vi "GetTACWindow.vi"(0 "Enum":enum16{"ini", "get", "quick"}(ring), 4 "auto":bool) -> (1 "TAC.Window (diff)":u16, 2 "Waveform Graph 2":refnum<vi>, 3 "Decays":u32[][](graph), 5 "TAC.Window (min)":u16, 6 "allchan?":bool, 7 "Cursor.Cursor Position:Cursor X":u16, 8 "Cursor.Cursor Position:Cursor X 2":u16, 9 "x-values":dbl[](array[numeric]) format="%.2f", 10 "ready?":bool)   [LabVIEW 2009]
uses:
  IMAGE Cluster 2.ctl
panel:
  out "rebinning":dbl
  out "TAC Range (ns)":sgl
  in  "ADC-Resolution":u16(ring) items=["8bit", "12bit", "4bit", "15bit"]
  in  "Ring":u8(ring)=1 items=["linear y-axis", "log y-axis"]
  out "Boolean 2":bool
  in  "TAC-Cube (for Spotfinder)":T1(ring)=enum."no Spotfinding"
  in  "OK Button":bool
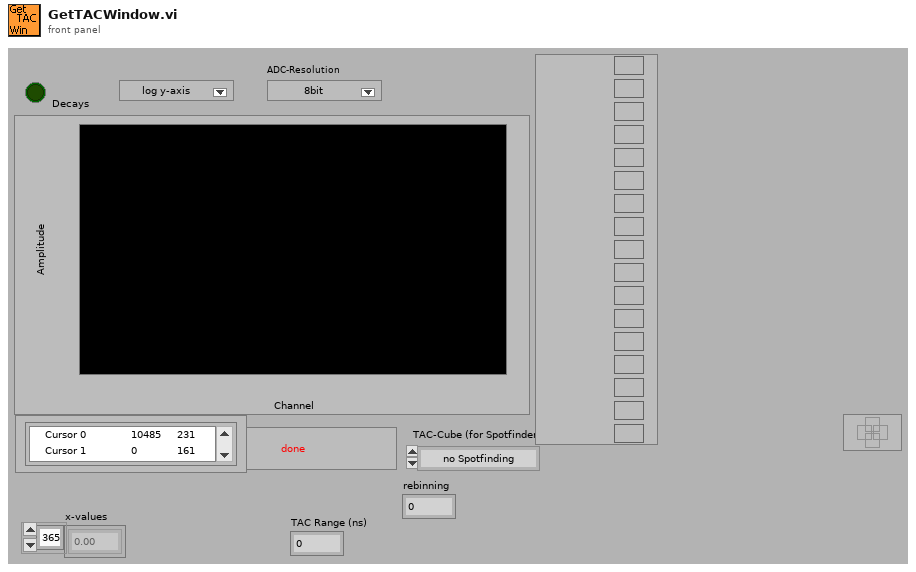
[diagram p1: front panel]
types:
  T1 = enum16{"1", "2", "3", "4", "5", "6", "7", "Sum", "no Spotfinding", "Separation"}
  T2 = typedef "IMAGE Cluster 2.ctl" = cluster{"decay":u16[][][][][], "sum of photons":u32[][][][]}
  T3 = typedef "FIFOSettings_BH.ctt" = cluster{"Measurement":cluster{"Binning (ms)":sgl, "External Trigger Condition":u16, "Stop Condition:":u16, "Stop Count":dbl, "Buffer Size (Photons)":u16, "No of Channels":u16, "Ext Latch Delay":i16}, "ADC":cluster{"Module":u16, "ADC Resolution":i32, "Dither Range":i16, "Count Increment":i16, "Macro Time Clock":i16}, "SYNC":cluster{"SYNC ZC Level (mV)":sgl, "SYNC Freq Divider":i16, "SYNC Holdoff (ns)":sgl, "SYNC Threshold (mV)":sgl}, "TAC":cluster{"TAC Range (ns)":sgl, "TAC Gain":i16, "TAC Offset (%)":sgl, "TAC Limit Low (%)":sgl, "TAC Limit High (%)":sgl}, "CFD":cluster{"CFD Limit Low (mV)":sgl, "CFD Limit High (mV)":sgl, "CFD ZC Level (mV)":sgl, "CFD Holdoff (ns)":sgl}}
  T4 = typedef "Settings.ctl" = cluster{"threshold":cluster{"max":u32, "min":u32}, "RGB or false color":bool, "16bit":bool, "log/lin axis":u16, "spotsize button":bool, "Pixelsize":u16, "autoscale x":bool, "autoscale y":bool, "correlation":bool, "ADC-Resolution":i32, "F2-lifetime":cluster{"display tau":bool, "display F2":bool, "Palette Number lifetime":enum32{"Gray", "Binary", "Gradient", "Rainbow", "Temperature"}, "Palette Number F2":enum32{"Gray", "Binary", "Gradient", "Rainbow", "Temperature"}, "max tau-Value":dbl, "min tau-Value":dbl, "max F2-Value":dbl, "min F2-Value":dbl}, "TAC-Window 1":u16, "TAC-Window 2":u16, "false color palette":cluster{"1":u32, "2":u32, "3":u32, "4":u32, "5":u32, "6":u32, "7":u32, "8":u32, "8 2":u32, "8 3":u32, "8 4":u32, "8 5":u32}, "rebinning":dbl}
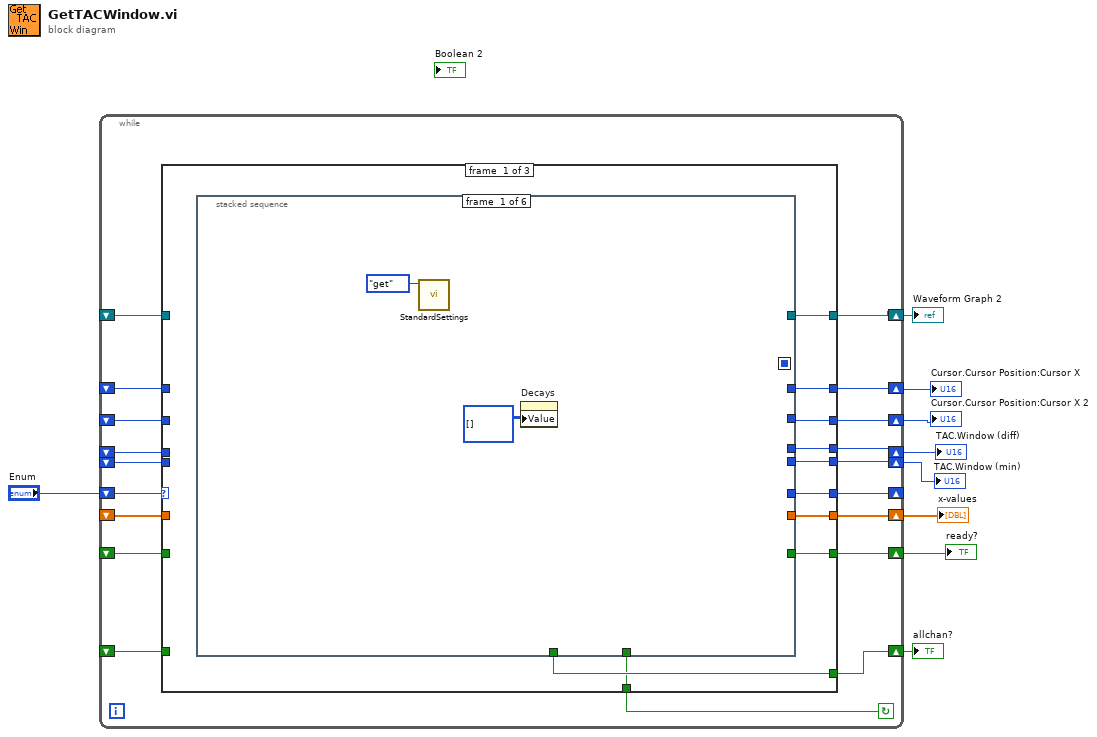
[diagram p0: block diagram]
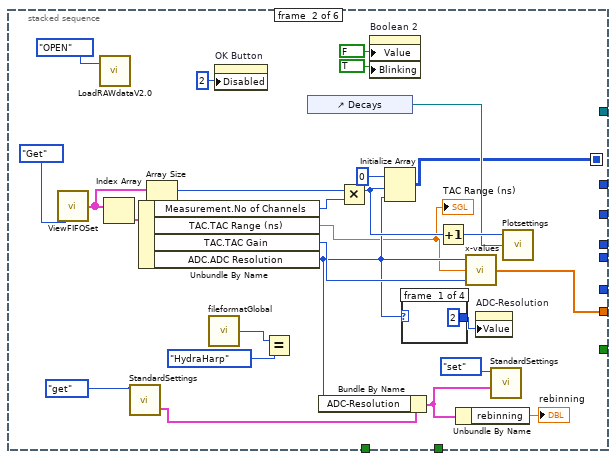
[diagram p2: hidden frame]
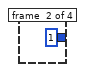
[diagram p3: hidden frame]
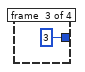
[diagram p4: hidden frame]
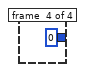
[diagram p5: hidden frame]
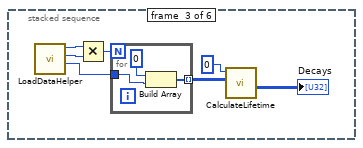
[diagram p6: hidden frame]
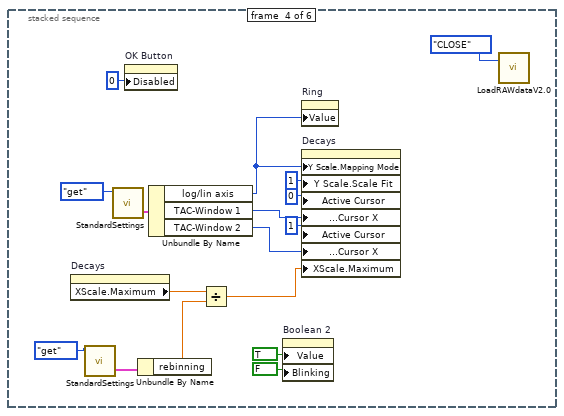
[diagram p7: hidden frame]
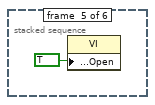
[diagram p8: hidden frame]
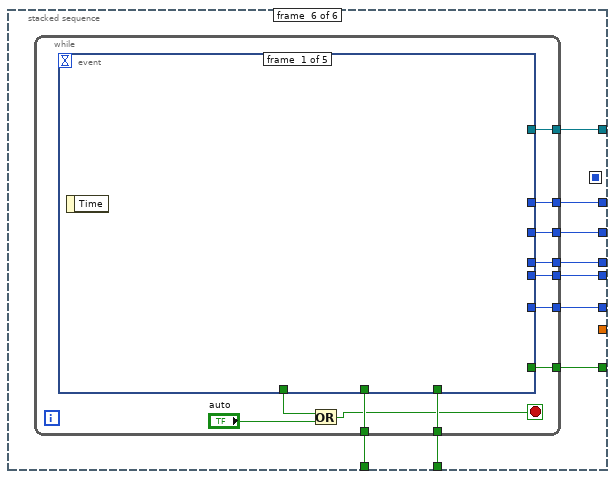
[diagram p9: hidden frame]
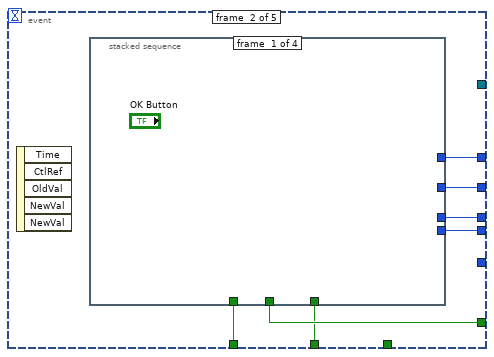
[diagram p10: hidden frame]
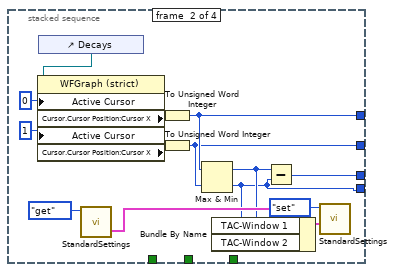
[diagram p11: hidden frame]
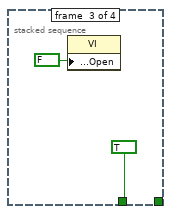
[diagram p12: hidden frame]
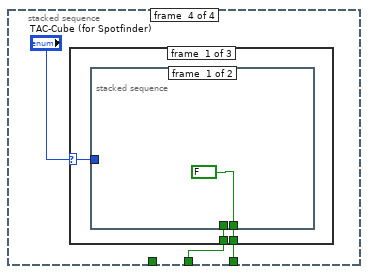
[diagram p13: hidden frame]
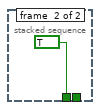
[diagram p14: hidden frame]
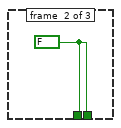
[diagram p15: hidden frame]
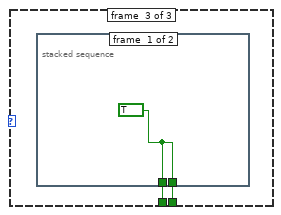
[diagram p16: hidden frame]
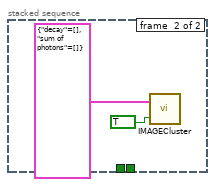
[diagram p17: hidden frame]
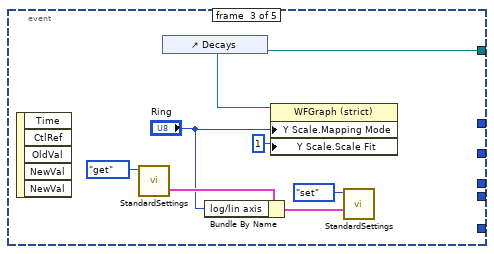
[diagram p18: hidden frame]
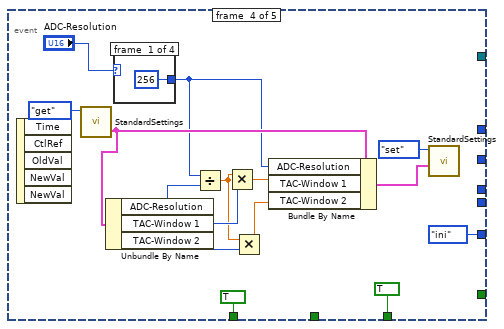
[diagram p19: hidden frame]
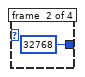
[diagram p20: hidden frame]
diagram:
  n1 = while {
    shift-right: [w28] -> w8
    shift-left: _ -> [w26]
    shift-right: [w27] -> w9
    shift-left: _ -> [w25]
    shift-right: [w24] -> w7
    shift-left: _ -> [w23]
    shift-right: [w21] -> w5
    shift-left: _ -> [w19]
    shift-right: [w22] -> w6
    shift-left: _ -> [w20]
    shift-right: [w13] -> w4
    shift-left: _ -> [w18]
    shift-right: [w17] -> w3
    shift-left: _ -> [w16]
    shift-right: [w15] -> w2
    shift-left: _ -> [w14]
    shift-right: [w10] -> _
    shift-left: "Enum" -> [w11]
    stop <- w12 continue-if-true
    n2 = case shown="\"ini\", Default" w11 {
      tunnel: [w38 w191 w205] -> w28
      tunnel: [w37 w190 w204] -> w27
      tunnel: w26 -> [_ w191 _]
      tunnel: w25 -> [_ w190 _]
      tunnel: [w36 w189 w193] -> w24
      tunnel: w23 -> [_ w189 _]
      tunnel: [w35 w188 w210] -> w22
      tunnel: [w34 w187 w211] -> w21
      tunnel: w20 -> [_ w188 w210]
      tunnel: w19 -> [_ w187 w211]
      tunnel: [w33 w186 w212] -> w13
      tunnel: w18 -> [_ w186 w212]
      tunnel: [w32 w185 w209] -> w17
      tunnel: w16 -> [_ w185 w209]
      tunnel: [w31 w184 w208] -> w15
      tunnel: w14 -> [_ w184 w208]
      tunnel: [w30 _ _] -> w12
      tunnel: [w29 _ _] -> w10
      frame #0 {
        n3 = stacked-sequence {
          seq-local: [_ w42 _ _ _ _] -> [_ _ _ _ _ _]
          tunnel: [_ _ _ _ _ w107] -> w38
          tunnel: [_ _ _ _ _ w106] -> w37
          tunnel: [_ w47 _ _ _ _] -> w36
          tunnel: [_ _ _ _ _ w105] -> w35
          tunnel: [_ _ _ _ _ w104] -> w34
          tunnel: [_ _ _ _ _ w103] -> w33
          tunnel: [_ _ _ _ _ w102] -> w32
          tunnel: [_ _ _ _ _ w101] -> w31
          tunnel: [_ _ _ _ _ w100] -> w30
          tunnel: [_ _ _ _ _ w99] -> w29
          frame #0 {
            n4 = call "StandardSettings.vi"("Enum"=enum16{"Load", "get", "Save", "set"}."get") -> ()  [unwired: 4 in, 1 out]
            n5 = property on="Decays" class="WFGraph (strict)"("Value"=u32[][] [] ("Waveform Graph")) -> ()  [unwired: 2 in, 2 out]
          }
          frame #1 {
            n6 = call "ViewFIFOSet.vi"("Enum"=enum16{"Display", "change", "Get", "Set"}."Get") -> ("FIFO Settings (Array)"=w54:T3[])  [unwired: 1 in]
            n7 = call "LoadRAWdataV2.0.vi"("action"=enum16{"OPEN", "READ", "CLOSE"}."OPEN" ("Enum")) -> ()  [unwired: 1 in, 2 out]
            n8 = Index Array(array=w54) -> (element=w55:T3)  [unwired: 1 in]
            n9 = call "StandardSettings.vi"("Enum"=enum16{"Load", "get", "Save", "set"}."get") -> ("StandardSettings"=w46:T4)  [unwired: 4 in]
            n10 = Unbundle By Name(w55) -> ("Measurement.No of Channels"=w53:u16, "TAC.TAC Range (ns)"=w41:sgl, "TAC.TAC Gain"=w61:i16, "ADC.ADC Resolution"=w50:i32)
            "TAC Range (ns)" <- w41
            n11 = Array Size(array=w54) -> (size(s)=w52:i32)
            n12 = call "fileformatGlobal.vi"() -> ("fileformat out"=w49:enum16{"Herty", "Ken", "SPC130", "HydraHarp"})  [unwired: 2 in]
            n13 = property on="OK Button" class="Boolean"("Disabled"=u8 2) -> ()  [unwired: 2 in, 2 out]
            n14 = Equal?(x=w49, y=enum16{"Herty", "Ken", "SPC130", "HydraHarp"}."HydraHarp") -> ()  [unwired: 1 out]
            n15 = control-ref of="Decays"() -> (w56:refnum<vi>)
            n16 = Bundle By Name(cluster=w46, "ADC-Resolution"=w50) -> (w44:T4)
            n17 = Multiply(x=w52, y=w53) -> (x*y=w51:i32)
            n18 = property on="Boolean 2" class="Boolean (strict)"("Value"=FALSE ("Boolean 2"), "Blinking"=TRUE) -> ()  [unwired: 2 in, 2 out]
            n19 = Initialize Array(u32 0 ("element"), w51, w50) -> (w42:u32[][])
            n20 = case shown="32768" w50 {
              tunnel: [u16 2 u16 1 u16 3 u16 0] -> w43
              frame #0 {
              }
              frame #1 {
              }
              frame #2 {
              }
              frame #3 {
              }
            }
            n21 = Increment(x=w51) -> (x+1=w58:i32)
            n22 = Unbundle By Name(w44) -> ("rebinning"=→"rebinning":dbl)
            n23 = call "x-values.vi"("TAC Gain"=w61, "TAC Rang [ns]"=w41, "No. Microchannel"=w50) -> ("Array"=w47:dbl[])
            n24 = property on="ADC-Resolution" class="Ring (strict)"("Value"=w43) -> ()  [unwired: 2 in, 2 out]
            n25 = call "StandardSettings.vi"("StandardSettings"=w44, "Enum"=enum16{"Load", "get", "Save", "set"}."set") -> ()  [unwired: 3 in, 1 out]
            n26 = call "Plotsettings.vi"("Decays 2"=w56, "No of Channels"=w58) -> ()  [unwired: 4 in]
          }
          frame #2 {
            n27 = call "LoadDataHelper.vi"() -> ("pixel per line"=w73:u32, "planes"=w74:u32, "lines"=w75:u32)  [unwired: 7 in, 2 out]
            n28 = Multiply(x=w75, y=w74) -> (x*y=w76:u32)
            n29 = for {
              N: w76 -> [_]
              tunnel: w73 -> [w79]
              tunnel: [w78] -> w72 mode=indexing
              n30 = Build Array(0 ("starting y-point"), w79) -> (w78:u32[])
            }
            n31 = call "CalculateLifetime.vi"("Pos Array"=w72, "starting y-point"=0) -> ("Decay"=→"Decays":u32[][])  [unwired: 5 in]
          }
          frame #3 {
            n32 = property on="Decays" class="WFGraph (strict)"() -> ("XScale.Maximum"=w85:dbl)  [unwired: 2 in, 2 out]
            n33 = call "StandardSettings.vi"("Enum"=enum16{"Load", "get", "Save", "set"}."get") -> ("StandardSettings"=w83:T4)  [unwired: 4 in]
            n34 = call "StandardSettings.vi"("Enum"=enum16{"Load", "get", "Save", "set"}."get") -> ("StandardSettings"=w92:T4)  [unwired: 4 in]
            n35 = property on="OK Button" class="Boolean"("Disabled"=u8 0) -> ()  [unwired: 2 in, 2 out]
            n36 = Unbundle By Name(w83) -> ("rebinning"=w82:dbl)
            n37 = Unbundle By Name(w92) -> ("log/lin axis"=w87:u16, "TAC-Window 1"=w89:u16, "TAC-Window 2"=w88:u16)
            n38 = Divide(x=w85, y=w82) -> (x/y=w81:dbl)
            n39 = property on="Boolean 2" class="Boolean (strict)"("Value"=TRUE ("Boolean 2"), "Blinking"=FALSE) -> ()  [unwired: 2 in, 2 out]
            n40 = property on="Ring" class="Ring (strict)"("Value"=w87) -> ()  [unwired: 2 in, 2 out]
            n41 = property on="Decays" class="WFGraph (strict)"("Y Scale.Mapping Mode"=w87, "Y Scale.Scale Fit"=u8 1, "Active Cursor"=u32 0, "Cursor.Cursor Position:Cursor X"=w89, "Active Cursor"=u32 1, "Cursor.Cursor Position:Cursor X"=w88, "XScale.Maximum"=w81) -> ()  [unwired: 2 in, 2 out]
            n42 = call "LoadRAWdataV2.0.vi"("action"=enum16{"OPEN", "READ", "CLOSE"}."CLOSE" ("Enum")) -> ()  [unwired: 1 in, 2 out]
          }
          frame #4 {
            n43 = property class="VI"("Front Panel Window:Open"=TRUE) -> ()  [unwired: 2 in, 2 out]
          }
          frame #5 {
            n44 = while {
              tunnel: [w119] -> w107
              tunnel: [w118] -> w106
              tunnel: [w117] -> w105
              tunnel: [w116] -> w104
              tunnel: [w115] -> w103
              tunnel: [w114] -> w102
              tunnel: [w113] -> w101
              tunnel: [w112] -> w100
              tunnel: [w111] -> w99
              stop <- w108 stop-if-true
              n45 = event shown="[1] \"OK Button\": Value Change" {
                selector: _ -> [_ _ _ _ _]
                dyn-events: _ -> [_ _ _ _ _]
                timeout: _ -> [_ _ _ _ _]
                tunnel: [_ w126 _ TRUE TRUE] -> w110
                tunnel: [_ w125 _ _ _] -> w119
                tunnel: [_ w124 _ _ _] -> w118
                tunnel: [_ w123 _ _ _] -> w117
                tunnel: [_ w122 _ _ _] -> w116
                tunnel: [_ w121 _ _ _] -> w115
                tunnel: [_ _ w163 _ _] -> w114
                tunnel: [_ w120 _ _ _] -> w113
                tunnel: [_ _ _ TRUE _] -> w112
                tunnel: [_ _ _ enum16{"ini", "get", "quick"}."ini" ("Enum") _] -> w111
                event #0 {
                  n46 = event-data() -> ()  [unwired: 1 in, 1 out]
                }
                event #1 {
                  n47 = event-data() -> ()  [unwired: 1 in, 5 out]
                  n48 = stacked-sequence {
                    tunnel: [_ _ TRUE _] -> w126
                    tunnel: [_ w130 _ _] -> w125
                    tunnel: [_ w129 _ _] -> w124
                    tunnel: [_ w136 _ _] -> w123
                    tunnel: [_ w127 _ _] -> w122
                    tunnel: [_ _ _ w144] -> w121
                    tunnel: [_ _ _ w143] -> w120
                    frame #0 {
                    }
                    frame #1 {
                      n49 = control-ref of="Decays"() -> (w135:refnum<vi>)
                      n50 = property class="WFGraph (strict)"(reference=w135, "Active Cursor"=u32 0, "Active Cursor"=u32 1) -> ("Cursor.Cursor Position:Cursor X"=w138:dbl, "Cursor.Cursor Position:Cursor X"=w137:dbl)  [unwired: 1 in, 2 out]
                      n51 = call "StandardSettings.vi"("Enum"=enum16{"Load", "get", "Save", "set"}."get") -> ("StandardSettings"=w132:T4)  [unwired: 4 in]
                      n52 = To Unsigned Word Integer(number=w138) -> (unsigned 16bit integer=w130:u16)
                      n53 = To Unsigned Word Integer(number=w137) -> (unsigned 16bit integer=w129:u16)
                      n54 = Max & Min(x=w130, y=w129) -> (max(x,y)=w128:u16, min(x,y)=w127:u16)
                      n55 = Bundle By Name(cluster=w132, "TAC-Window 1"=w128, "TAC-Window 2"=w127) -> (w131:T4)
                      n56 = Subtract(x=w128, y=w127) -> (x-y=w136:u16)
                      n57 = call "StandardSettings.vi"("StandardSettings"=w131, "Enum"=enum16{"Load", "get", "Save", "set"}."set") -> ()  [unwired: 3 in, 1 out]
                    }
                    frame #2 {
                      n58 = property class="VI"("Front Panel Window:Open"=FALSE) -> ()  [unwired: 2 in, 2 out]
                    }
                    frame #3 {
                      n59 = case shown="\"1\", Default" "TAC-Cube (for Spotfinder)" {
                        selector: "TAC-Cube (for Spotfinder)" -> [w148 _ _]
                        tunnel: [w147 w151 w153] -> w144
                        tunnel: [w146 w151 w152] -> w143
                        frame #0 {
                          n60 = stacked-sequence {
                            tunnel: w148 -> [_ _]
                            tunnel: [_ TRUE] -> w147
                            tunnel: [FALSE ("allchan?") _] -> w146
                            frame #0 {
                            }
                            frame #1 {
                            }
                          }
                        }
                        frame #1 {
                          w151 = FALSE
                        }
                        frame #2 {
                          n61 = stacked-sequence {
                            tunnel: [w154 _] -> w153
                            tunnel: [w154 _] -> w152
                            frame #0 {
                              w154 = TRUE ("allchan?")
                            }
                            frame #1 {
                              n62 = call "IMAGECluster.vi"("set?"=TRUE, "IMAGE Cluster in"=T2 {"decay"=[], "sum of photons"=[]} ("IMAGE Cluster (input)")) -> ()  [unwired: 1 out]
                            }
                          }
                        }
                      }
                    }
                  }
                }
                event #2 {
                  n63 = event-data() -> ()  [unwired: 1 in, 5 out]
                  n64 = call "StandardSettings.vi"("Enum"=enum16{"Load", "get", "Save", "set"}."get") -> ("StandardSettings"=w160:T4)  [unwired: 4 in]
                  n65 = control-ref of="Decays"() -> (w163:refnum<vi>)
                  n66 = Bundle By Name(cluster=w160, "log/lin axis"="Ring") -> (w159:T4)
                  n67 = property class="WFGraph (strict)"(reference=w163, "Y Scale.Mapping Mode"="Ring", "Y Scale.Scale Fit"=u8 1) -> ()  [unwired: 1 in, 2 out]
                  n68 = call "StandardSettings.vi"("StandardSettings"=w159, "Enum"=enum16{"Load", "get", "Save", "set"}."set") -> ()  [unwired: 3 in, 1 out]
                }
                event #3 {
                  n69 = event-data() -> ()  [unwired: 1 in, 5 out]
                  n70 = call "StandardSettings.vi"("Enum"=enum16{"Load", "get", "Save", "set"}."get") -> ("StandardSettings"=w174:T4)  [unwired: 4 in]
                  n71 = Unbundle By Name(w174) -> ("ADC-Resolution"=w164:i32, "TAC-Window 1"=w169:u16, "TAC-Window 2"=w170:u16)
                  n72 = case shown="2" "ADC-Resolution" {
                    tunnel: [256 32768 4096 128] -> w165
                    frame #0 {
                    }
                    frame #1 {
                    }
                    frame #2 {
                    }
                    frame #3 {
                    }
                  }
                  n73 = Divide(x=w165, y=w164) -> (x/y=w168:dbl)
                  n74 = Multiply(x=w168, y=w169) -> (x*y=w167:dbl)
                  n75 = Multiply(x=w168, y=w170) -> (x*y=w166:dbl)
                  n76 = Bundle By Name(cluster=w174, "ADC-Resolution"=w165, "TAC-Window 1"=w167, "TAC-Window 2"=w166) -> (w173:T4)
                  n77 = call "StandardSettings.vi"("StandardSettings"=w173, "Enum"=enum16{"Load", "get", "Save", "set"}."set") -> ()  [unwired: 3 in, 1 out]
                }
                event #4 {
                  n78 = event-data() -> ()  [unwired: 1 in, 3 out]
                  n79 = event-data() -> ()  [unwired: 2 in, 1 out]
                }
              }
              n80 = Or(x=w110, y="auto") -> (x .or. y?=w108:bool)
            }
          }
        }
      }
      frame #1 {
      }
      frame #2 {
        n81 = call "ViewFIFOSet.vi"("Enum"=enum16{"Display", "change", "Get", "Set"}."Get") -> ("FIFO Settings (Array)"=w213:T3[])  [unwired: 1 in]
        n82 = call "StandardSettings.vi"("Enum"=enum16{"Load", "get", "Save", "set"}."get") -> ("StandardSettings"=w206:T4)  [unwired: 4 in]
        n83 = Index Array(array=w213) -> (element=w192:T3)  [unwired: 1 in]
        n84 = Unbundle By Name(w206) -> ("TAC-Window 1"=w205:u16, "TAC-Window 2"=w204:u16, "ADC-Resolution"=w196:i32)
        n85 = Unbundle By Name(w192) -> ("ADC.ADC Resolution"=w195:i32, "TAC.TAC Range (ns)"=w197:sgl, "TAC.TAC Gain"=w198:i16)
        n86 = Not Equal To 0?(x=w195) -> (x != 0?=w202:bool)
        n87 = Select(t=4096, s=w202, f=256) -> (s? t:f=w194:i32)
        n88 = Greater?(x=w194, y=w196) -> (0:w200:bool)
        n89 = Select(t=w196, s=w200, f=w194) -> (s? t:f=w199:i32)
        n90 = call "x-values.vi"("TAC Gain"=w198, "TAC Rang [ns]"=w197, "No. Microchannel"=w199) -> ("Array"=w193:dbl[])
      }
    }
  }
  "Cursor.Cursor Position:Cursor X 2" <- w9
  "Cursor.Cursor Position:Cursor X" <- w8
  "x-values" <- w7
  "TAC.Window (diff)" <- w6
  "TAC.Window (min)" <- w5
  "ready?" <- w4
  "Waveform Graph 2" <- w3
  "allchan?" <- w2
